vi "Modify User Details.vi"(8 "error in":errorcluster, 9 "USER DATABASE":i32(listbox), 10 "Path":path=path "D:/SVN/USERS/SUBASREE/pass manager/user_database.xls") -> (0 "error out":errorcluster)   [LabVIEW 2015]
uses:
  <vilib>/Utility/file.llb/Write Delimited Spreadsheet (string).vi
  <vilib>/Utility/file.llb/Read Delimited Spreadsheet (string).vi
panel:
  in  "hide(F)/show(T)":bool
  in  "Password":string
  out "User Name":string
  in  "Designation":u16(ring) items=["Select the Designation", "Operator", "Supevisor", "Admin"]
  in  "OK":bool
  in  "Cancel":bool
  # "Modify User Credential"
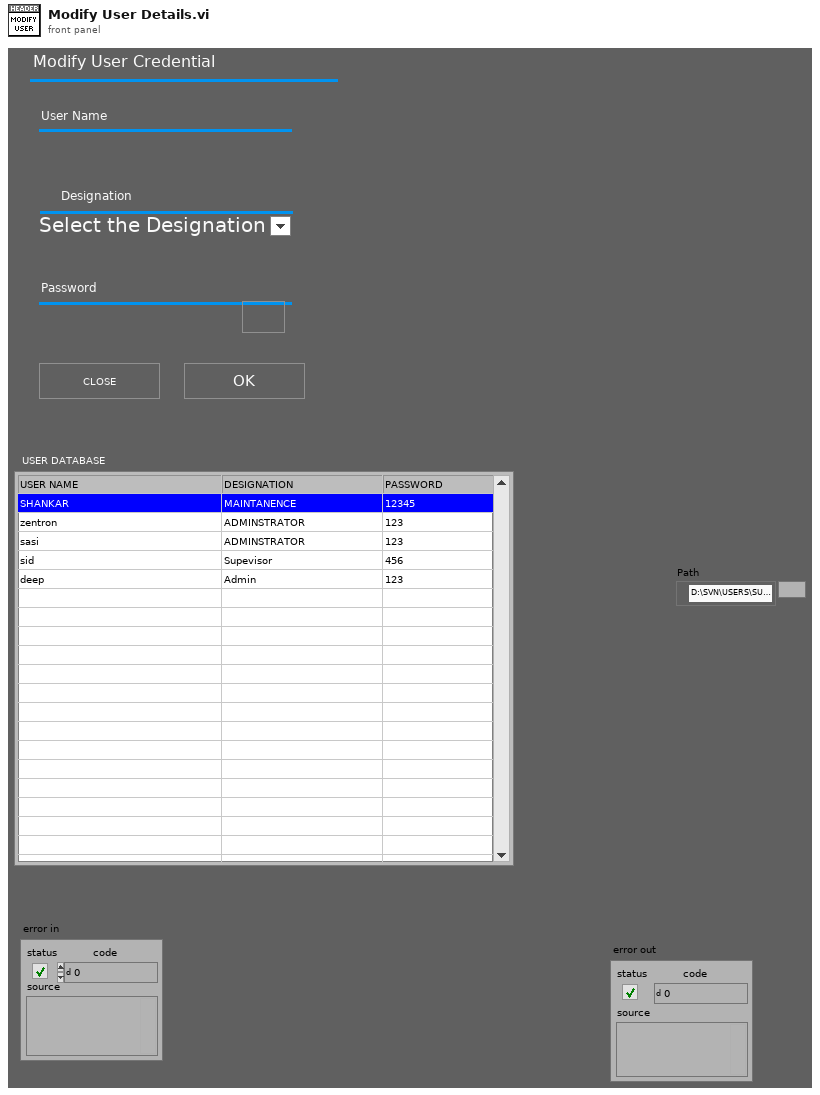
[diagram p1: front panel]
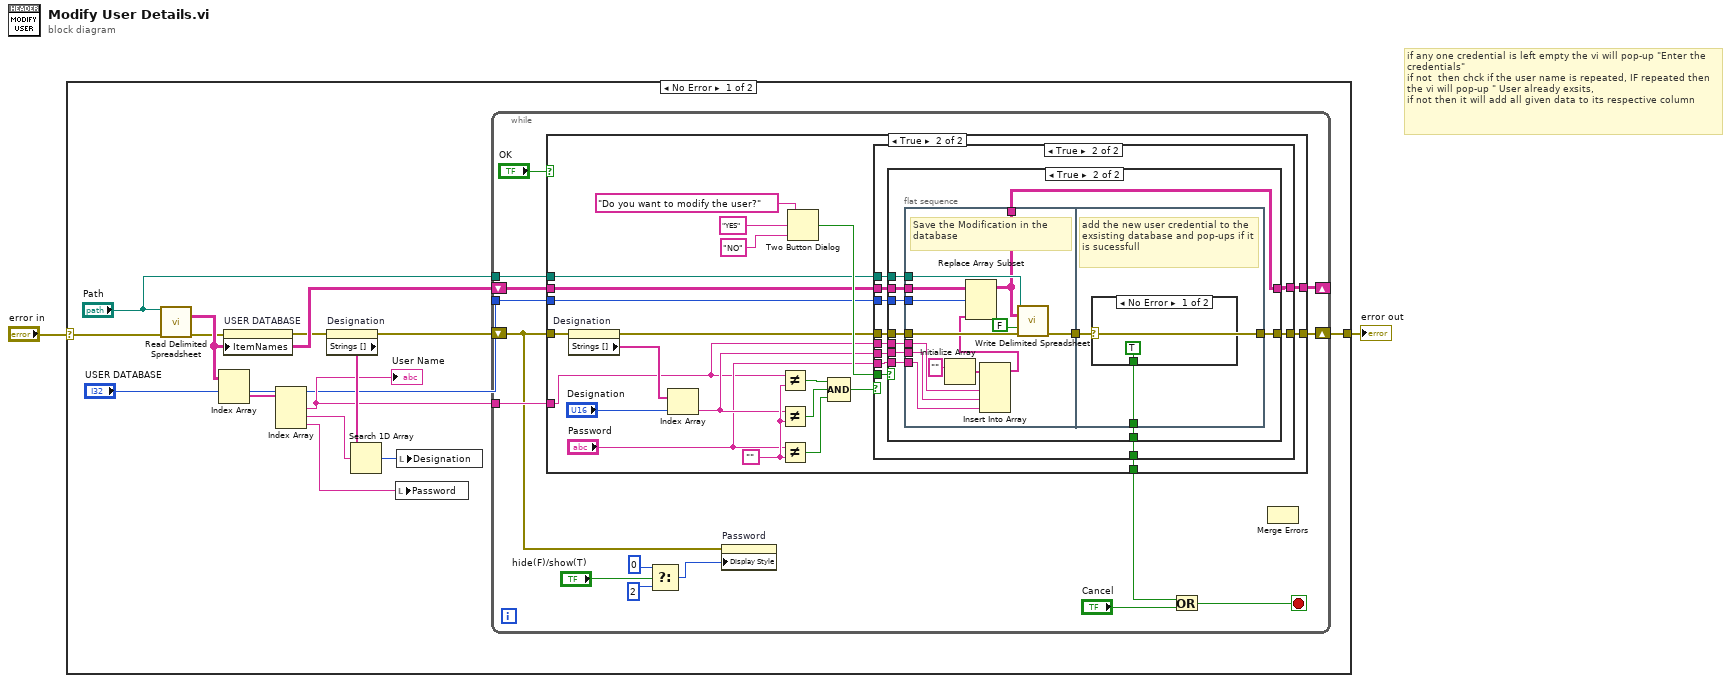
[diagram p0: block diagram]
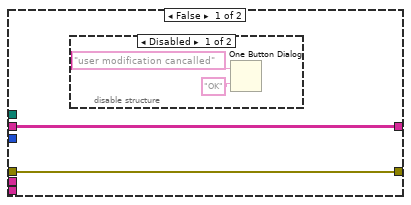
[diagram p4: hidden frame]
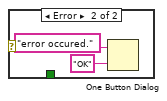
[diagram p6: hidden frame]
diagram:
  # "if any one credential is left empty the vi will pop-up \"Enter the credentials\" \nif not  then chck if the user name is repeated, IF repeated then the vi will pop-up \" User already exsits,\nif not then it will add all given data to its respective column"
  n1 = case shown="No Error" "error in" {
    selector: "error in" -> [w3 w102]
    tunnel: [w4 w102] -> w1
    frame No Error {
      n2 = call-poly <vilib>:"Read Delimited Spreadsheet.vi"("file path (dialog if empty)"="Path", "error in (no error)"=w3) -> ("all rows"=w10:string[][], "error out"=w8:errorcluster)  [unwired: 8 in, 4 out]
      n3 = Index Array(array=w10, index (row)="USER DATABASE") -> (element=w16:string[])  [unwired: 1 in]
      n4 = property on="USER DATABASE" class="MCListbox (strict)"(error in=w8, "ItemNames"=w10) -> (error out=w7:errorcluster)  [unwired: 1 in, 1 out]
      n5 = Index Array(array=w16) -> (element #1=w9:string, element #2=w14:string, element #3=w12:string)  [unwired: 3 in]
      "User Name" <- w9
      n6 = property on="Designation" class="Ring (strict)"(error in=w7) -> (error out=w6:errorcluster, "Strings []"=w15:string[])  [unwired: 1 in, 1 out]
      n7 = Search 1D Array(1D array=w15, element=w14) -> (index of element=w13:i32)  [unwired: 1 in]
      n8 = local write "Password"(w12) -> ()
      n9 = local write "Designation"(w13) -> ()
      n10 = while {
        tunnel: w9 -> [w28]
        tunnel: "Path" -> [w31]
        shift-right: [w27] -> _
        shift-left: w10 -> [w30]
        tunnel: "USER DATABASE" -> [w29]
        shift-right: [w25] -> w4
        shift-left: w6 -> [w21]
        stop <- w22 stop-if-true
        n11 = case shown="True" "OK" {
          tunnel: w31 -> [_ w45]
          tunnel: w30 -> [w33 w44]
          tunnel: w29 -> [_ w43]
          tunnel: w28 -> [_ w35]
          tunnel: [w33 w40] -> w27
          tunnel: w21 -> [w32 w38]
          tunnel: [w32 w36] -> w25
          tunnel: [_ w34] -> w24
          frame False {
          }
          frame True {
            w46 = ""
            n12 = property on="Designation" class="Ring (strict)"(error in=w38) -> (error out=w37:errorcluster, "Strings []"=w50:string[])  [unwired: 1 in, 1 out]
            n13 = Index Array(array=w50, index="Designation") -> (element=w42:string)
            n14 = Not Equal?(x=w35, y=w46) -> (x != y?=w47:bool)
            n15 = Not Equal?(x=w42, y=w46) -> (x != y?=w48:bool)
            n16 = Not Equal?(x="Password", y=w46) -> (x != y?=w49:bool)
            n17 = Two Button Dialog(message="Do you want to modify the user?", 1:"NO" ("button name (\"OK\")"), 2:"YES" ("T button name (\"OK\")")) -> (T button?=w52:bool)
            n18 = Compound Arithmetic op=AND(w47, w48, w49) -> (w39:bool)
            n19 = case shown="True" w39 {
              tunnel: w44 -> [w57 w68]
              tunnel: w45 -> [_ w67]
              tunnel: w42 -> [_ w66]
              tunnel: w35 -> [_ w65]
              tunnel: w43 -> [_ w64]
              tunnel: w52 -> [_ w63]
              tunnel: [w57 w62] -> w40
              tunnel: "Password" -> [_ w61]
              tunnel: w37 -> [w56 w60]
              tunnel: [w56 w59] -> w36
              tunnel: [_ w58] -> w34
              frame False {
              }
              frame True {
                n20 = case shown="True" w63 {
                  tunnel: w68 -> [w70 w83]
                  tunnel: w67 -> [_ w82]
                  tunnel: w61 -> [_ w81]
                  tunnel: w66 -> [_ w80]
                  tunnel: w65 -> [_ w79]
                  tunnel: w64 -> [_ w77]
                  tunnel: [w70 w76] -> w62
                  tunnel: w60 -> [w69 w75]
                  tunnel: [w69 w74] -> w59
                  tunnel: [_ w73] -> w58
                  frame False {
                    n21 = disable-structure shown="Disabled" {
                      frame Disabled {
                        n22 = One Button Dialog(message="user modification cancalled", button name ("OK")="OK") -> ()  [unwired: 1 out]
                      }
                      frame Enabled {
                      }
                    }
                  }
                  frame True {
                    n23 = flat-sequence {
                      tunnel: w83 -> [w96]
                      tunnel: w82 -> [w95]
                      tunnel: w81 -> [w85]
                      tunnel: w80 -> [w86]
                      tunnel: w79 -> [w87]
                      tunnel: [w94] -> w78
                      tunnel: w77 -> [w93]
                      tunnel: [w91] -> w76
                      tunnel: w75 -> [w90]
                      tunnel: w78 -> [w98]
                      tunnel: [w98] -> w74
                      tunnel: [w97] -> w73
                      frame #0 {
                        # "Save the Modification in the database"
                        n24 = Initialize Array("") -> (w88:string[])  [unwired: 1 in]
                        n25 = Insert Into Array(array=w88, new element #1=w87, new element #2=w86, new element #3=w85) -> (w84:string[])  [unwired: 1 in]
                        n26 = Replace Array Subset(array=w96, new element=w84, index (row)=w93) -> (w91:string[][])  [unwired: 1 in]
                        n27 = call-poly <vilib>:"Write Delimited Spreadsheet.vi"("file path (dialog if empty)"=w95, "2D data"=w91, "append to file? (F)"=FALSE, "error in (no error)"=w90) -> ("error out"=w94:errorcluster)  [unwired: 10 in, 1 out]
                      }
                      frame #1 {
                        # "add the new user credential to the exsisting database and pop-ups if it is sucessfull"
                        n28 = case shown="No Error" w98 {
                          tunnel: [TRUE _] -> w97
                          frame No Error {
                          }
                          frame Error {
                            n29 = One Button Dialog(message="error occured.", button name ("OK")="OK") -> ()  [unwired: 1 out]
                          }
                        }
                      }
                    }
                  }
                }
              }
            }
          }
        }
        n30 = Select(t=u32 0 ("Display Style"), s="hide(F)/show(T)", f=u32 2) -> (s? t:f=w17:u32)
        n31 = property on="Password" class="Str"(error in=w21, "Display Style"=w17) -> ()  [unwired: 1 in, 2 out]
        n32 = Or(x=w24, y="Cancel") -> (x .or. y?=w22:bool)
        n33 = Merge Errors() -> ()  [unwired: 2 in, 1 out]
      }
    }
    frame Error {
    }
  }
  "error out" <- w1
